vi "StringRemoveExample-LV2012.vi"() -> ()   [LabVIEW 2012]
uses:
  <vilib>/Utility/file.llb/Read From Spreadsheet File (string).vi
panel:
  in  "Tab Control":enum32{"String Control", "File"}(tab)
  in  "all rows":string[][](array[string])
  in  "file path (use dialog)":path
  in  "Characters to remove \n(\\code display default)":string="\u0000"
  out "Strings":string[][](array[string])
  out "Output array":dbl[][](array[numeric])
  # "Select the \"File\" tab if you'd like to remove the strings from a 2-D array from file.\nSelect the \"String control\" tab if you'd like to test this VI with your string."
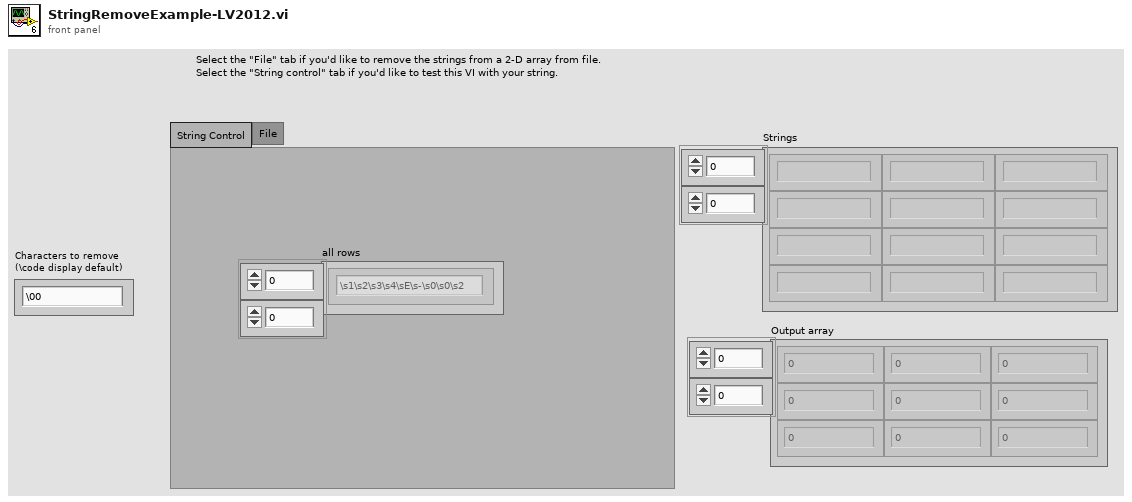
[diagram p1: front panel]
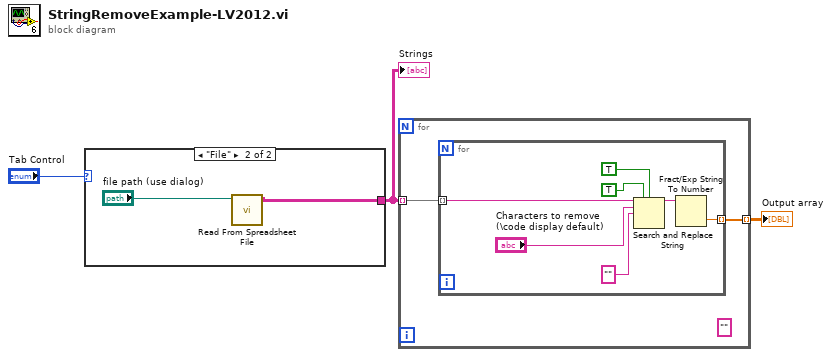
[diagram p0: block diagram]
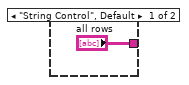
[diagram p2: hidden frame]
diagram:
  n1 = case shown="\"File\"" "Tab Control" {
    tunnel: ["all rows" w5] -> w3
    frame "String Control", Default {
    }
    frame "File" {
      n2 = call-poly <vilib>:"Read From Spreadsheet File.vi"("file path (dialog if empty)"="file path (use dialog)") -> ("all rows"=w5:string[][])  [unwired: 6 in, 4 out]
    }
  }
  "Strings" <- w3
  n3 = for {
    tunnel: [w8] -> w2 mode=indexing
    tunnel: w3 -> [w7] mode=indexing
    (unwired) "" ("element")
    n4 = for {
      tunnel: [w15] -> w8 mode=indexing
      tunnel: w7 -> [w9] mode=indexing
      n5 = Search and Replace String(replace all?=TRUE ("replace all? (F)"), case sensitive?=TRUE ("ignore case? (F)"), input string=w9, search string="Characters to remove \n(\\code display default)", replace string="" ("replace string (\"\")")) -> (result string=w10:string)  [unwired: 3 in, 3 out]
      n6 = Fract/Exp String To Number(string=w10) -> (number=w15:dbl)  [unwired: 3 in, 1 out]
    }
  }
  "Output array" <- w2
